vi "TestRole.vi"(8 "error in (no error)":errorcluster, 9 "Game in":refnum<class "Game.lvclass">, 10 "Robot":refnum<class "Robot.lvclass">, 11 "TestRole in":refnum<class "TestRole.lvclass">) -> (0 "error out":errorcluster, 1 "Game out":refnum<class "Game.lvclass">, 2 "Robot out":refnum<class "Robot.lvclass">, 3 "TestRole out":refnum<class "TestRole.lvclass">)   [LabVIEW 2023, in "TestRole.lvclass"]
uses:
  TestRole.lvclass
  C:/Users/ebert/Desktop/roboime/SSL_AI/Role_class/Role.lvclass
  Robot_class/Robot.lvclass
  Game_class/Game.lvclass
  Role_class/Role.lvclass/Role.ctl
  TestTactic_class/States.ctl
  Tacticbook_class/Tacticbook.lvclass/Tacticbook.ctl
  TestTactic_class/TestTactic.lvclass/TestTactic.ctl
  Tacticbook_class/Read TestTactic.vi
  TestTactic_class/Read States.vi
  Tacticbook_class/Write TestTactic.vi
  Role_class/Read Tacticbook.vi
  Role_class/Read tactic_index.vi
  Role_class/Write Tacticbook.vi
  Role_class/Write tactic_index.vi
  Role_class/Read RobotRef.vi
  Tacticbook_class/Tacticbook.lvclass
  TestTactic_class/TestTactic.lvclass
  TestRole.lvclass/TestRole.ctl
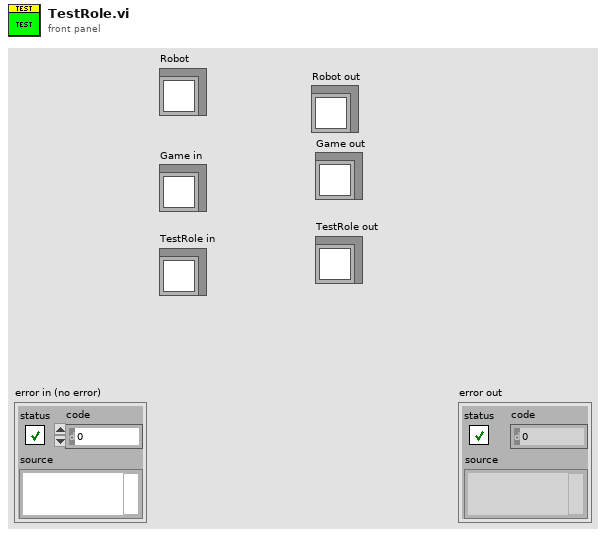
[diagram p1: front panel]
types:
  T1 = typedef "States.ctl" = enum16{"State 1", "Exit"}
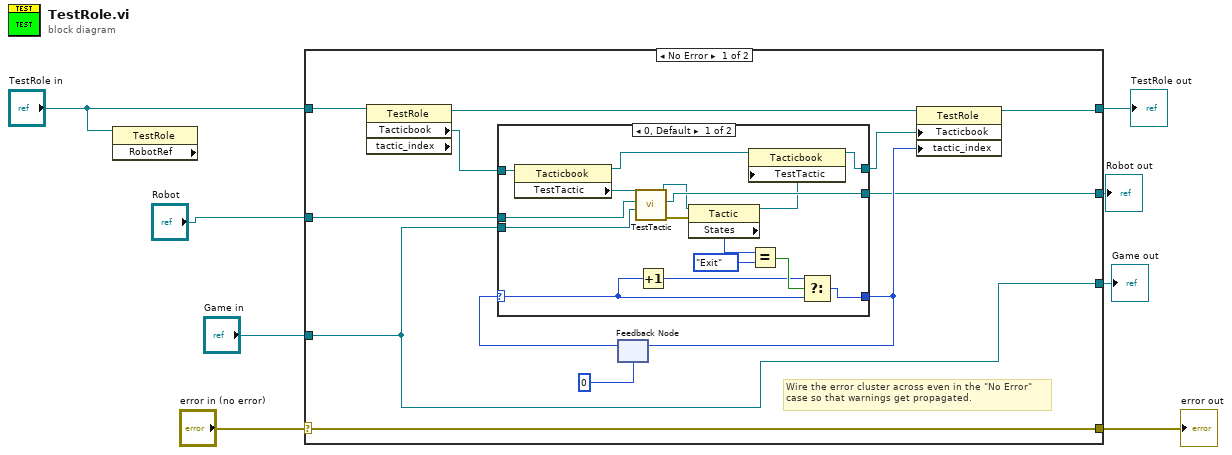
[diagram p0: block diagram]
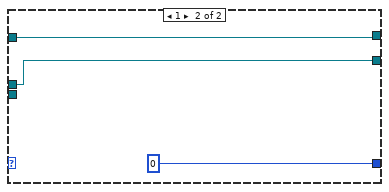
[diagram p2: hidden frame]
diagram:
  n1 = property class="TestRole" props=["RobotRef"](reference="TestRole in") -> ()  [unwired: 1 in, 3 out]
  n2 = case shown="No Error" "error in (no error)" {
    selector: "error in (no error)" -> [w20 w43]
    tunnel: [w20 w43] -> w7
    tunnel: [w18 w42] -> w6
    tunnel: "TestRole in" -> [w19 w42]
    tunnel: "Robot" -> [w12 w41]
    tunnel: [w11 w41] -> w5
    tunnel: [w9 w40] -> w4
    tunnel: "Game in" -> [w9 w40]
    frame No Error {
      # "Wire the error cluster across even in the \"No Error\"\ncase so that warnings get propagated."
      n3 = property class="TestRole" props=["Tacticbook", "tactic_index"](reference=w19) -> (reference out=w17:refnum<class "TestRole.lvclass">, "Tacticbook"=w14:refnum<class "Tacticbook.lvclass">)  [unwired: 1 in, 2 out]
      n4 = feedback #1(0) -> (w15:i32)
      n5 = case shown="0, Default" w15 {
        selector: w15 -> [w26 _]
        tunnel: [w27 0] -> w13
        tunnel: w14 -> [w36 w37]
        tunnel: w12 -> [w34 w39]
        tunnel: [w33 w39] -> w11
        tunnel: [w22 w37] -> w10
        tunnel: w9 -> [w21 _]
        frame 0, Default {
          n6 = property class="Tacticbook"(reference=w36) -> (reference out=w24:refnum<class "Tacticbook.lvclass">, "TestTactic"=w35:refnum<class "TestTactic.lvclass">)  [unwired: 1 in, 1 out]
          n7 = call-dynamic "TestTactic.vi"("Game in"=w21, "Robot"=w34, "Tactic in"=w35) -> ("error out"=w32:errorcluster, "Robot out"=w33:refnum<class "Robot.lvclass">, "Tactic out"=w31:refnum<class "TestTactic.lvclass">)  [unwired: 6 in]
          n8 = Increment(x=w26) -> (x+1=w25:i32)
          n9 = property class="Tactic"(reference=w31, error in=w32) -> (reference out=w23:refnum<class "TestTactic.lvclass">, "States"=w30:T1)  [unwired: 1 out]
          n10 = property class="Tacticbook"(reference=w24, "TestTactic"=w23) -> (reference out=w22:refnum<class "Tacticbook.lvclass">)  [unwired: 1 in, 1 out]
          n11 = Equal?(x=w30, y=States."Exit") -> (x = y?=w28:bool)
          n12 = Select(t=w25, s=w28, f=w26) -> (s? t:f=w27:i32)
        }
        frame 1 {
        }
      }
      n13 = feedback-in #1(w13) -> ()
      n14 = property class="TestRole"(reference=w17, "Tacticbook"=w10, "tactic_index"=w13) -> (reference out=w18:refnum<class "TestRole.lvclass">)  [unwired: 1 in, 1 out]
    }
    frame Error {
    }
  }
  "error out" <- w7
  "TestRole out" <- w6
  "Robot out" <- w5
  "Game out" <- w4
